vi "ATF_PUMP_PID_screen_V1.0.vi"() -> ()   [LabVIEW 2022 SP3]
panel:
  out "Countdown Timer (CDT)":dbl format="T%<+%H:%M:%S%3u>t"
  out "Date":timestamp format="%<%d/%m/%Y>T"
  in  "Close":bool
  in  "Screen No":dbl
  out "Indian Standard Time (IST)":timestamp format="%<%H:%M:%S%2u>T"
  out "B_AT_PV_19_HSS":bool
  out "B_AT_PV_19":bool caption="Boolean"
  out "B_AT_PV_18_HSS":bool
  out "B_AT_PV_18":bool caption="Boolean"
  out "B_AT_PV_16_HSS":bool
  out "B_AT_PV_16":bool caption="Boolean"
  out "B_AT_PV_14_HSS":bool
  out "B_AT_PV_14":bool caption="Boolean"
  out "B_AT_PV_12_HSS":bool
  out "B_AT_PV_12":bool caption="Boolean"
  out "B_AT_PV_10_HSS":bool
  out "B_AT_PV_10":bool caption="Boolean"
  out "B_AT_PV_08_HSS":bool
  out "B_AT_PV_08":bool caption="Boolean"
  out "B_AT_PV_06_HSS":bool
  out "B_AT_PV_06":bool caption="Boolean"
  out "B_AT_PV_04_HSS":bool
  out "B_AT_PV_04":bool caption="Boolean"
  out "B_AT_PV_02_HSS":bool
  out "B_AT_PV_02":bool caption="Boolean"
  out "B_AT_PV_17_HSS":bool
  out "B_AT_PV_17":bool caption="Boolean"
  out "B_AT_PV_15_HSS":bool
  out "B_AT_PV_15":bool caption="Boolean"
  out "B_AT_PV_13_HSS":bool
  out "B_AT_PV_13":bool caption="Boolean"
  out "B_AT_PV_11_HSS":bool
  out "B_AT_PV_11":bool caption="Boolean"
  out "B_AT_PV_09_HSS":bool
  out "B_AT_PV_09":bool caption="Boolean"
  out "B_AT_PV_07_HSS":bool
  out "B_AT_PV_07":bool caption="Boolean"
  out "B_AT_PV_05_HSS":bool
  out "B_AT_PV_05":bool caption="Boolean"
  out "B_AT_PV_03_HSS":bool
  out "B_AT_PV_03":bool caption="Boolean"
  out "B_AT_PV_01_HSS":bool
  out "B_AT_PV_01":bool caption="Boolean"
  out "S_PT_19":dbl format="%.2f bar"
  out "S_RTD_19":dbl format="%.2f bar"
  out "D_PT_19":dbl format="%.2f bar"
  out "D_RTD_19":dbl format="%.2f bar"
  out "S_PT_16":dbl format="%.2f bar"
  out "S_RTD_16":dbl format="%.2f bar"
  out "D_PT_16":dbl format="%.2f bar"
  out "D_RTD_16":dbl format="%.2f bar"
  out "S_PT_15":dbl format="%.2f bar"
  out "S_RTD_15":dbl format="%.2f bar"
  out "D_PT_15":dbl format="%.2f bar"
  out "D_RTD_15":dbl format="%.2f bar"
  out "S_PT_12":dbl format="%.2f bar"
  out "S_RTD_12":dbl format="%.2f bar"
  out "D_PT_12":dbl format="%.2f bar"
  out "D_RTD_12":dbl format="%.2f bar"
  out "S_PT_11":dbl format="%.2f bar"
  out "S_RTD_11":dbl format="%.2f bar"
  out "D_PT_11":dbl format="%.2f bar"
  out "D_RTD_11":dbl format="%.2f bar"
  out "S_PT_18":dbl format="%.2f bar"
  out "S_RTD_18":dbl format="%.2f bar"
  out "D_PT_18":dbl format="%.2f bar"
  out "D_RTD_18":dbl format="%.2f bar"
  out "S_PT_14":dbl format="%.2f bar"
  out "S_RTD_14":dbl format="%.2f bar"
  out "D_PT_14":dbl format="%.2f bar"
  out "D_RTD_14":dbl format="%.2f bar"
  out "S_PT_10":dbl format="%.2f bar"
  out "S_RTD_10":dbl format="%.2f bar"
  out "D_PT_10":dbl format="%.2f bar"
  out "D_RTD_10":dbl format="%.2f bar"
  out "S_PT_17":dbl format="%.2f bar"
  out "S_RTD_17":dbl format="%.2f bar"
  out "D_PT_17":dbl format="%.2f bar"
  out "D_RTD_17":dbl format="%.2f bar"
  out "S_PT_13":dbl format="%.2f bar"
  out "S_RTD_13":dbl format="%.2f bar"
  out "D_PT_13":dbl format="%.2f bar"
  out "D_RTD_13":dbl format="%.2f bar"
  out "S_PT_09":dbl format="%.2f bar"
  out "S_RTD_09":dbl format="%.2f bar"
  out "D_PT_09":dbl format="%.2f bar"
  out "D_RTD_09":dbl format="%.2f bar"
  out "S_PT_08":dbl format="%.2f bar"
  out "S_RTD_08":dbl format="%.2f bar"
  out "D_PT_08":dbl format="%.2f bar"
  out "D_RTD_08":dbl format="%.2f bar"
  out "S_PT_07":dbl format="%.2f bar"
  out "S_RTD_07":dbl format="%.2f bar"
  out "D_PT_07":dbl format="%.2f bar"
  out "D_RTD_07":dbl format="%.2f bar"
  out "S_PT_06":dbl format="%.2f bar"
  out "S_RTD_06":dbl format="%.2f bar"
  out "D_PT_06":dbl format="%.2f bar"
  out "D_RTD_06":dbl format="%.2f bar"
  out "S_PT_05":dbl format="%.2f bar"
  out "S_RTD_05":dbl format="%.2f bar"
  out "D_PT_05":dbl format="%.2f bar"
  out "D_RTD_05":dbl format="%.2f bar"
  out "S_PT_04":dbl format="%.2f bar"
  out "S_RTD_04":dbl format="%.2f bar"
  out "D_PT_04":dbl format="%.2f bar"
  out "D_RTD_04":dbl format="%.2f bar"
  out "S_PT_03":dbl format="%.2f bar"
  out "S_RTD_03":dbl format="%.2f bar"
  out "D_PT_03":dbl format="%.2f bar"
  out "D_RTD_03":dbl format="%.2f bar"
  out "S_PT_02":dbl format="%.2f bar"
  out "S_RTD_02":dbl format="%.2f bar"
  out "D_PT_02":dbl format="%.2f bar"
  out "D_RTD_02":dbl format="%.2f bar"
  out "S_PT_01":dbl format="%.2f bar"
  out "S_RTD_01":dbl format="%.2f bar"
  out "D_PT_01":dbl format="%.2f bar"
  out "D_RTD_01":dbl format="%.2f bar"
  out "B_AT_T_04":dbl format="%.2f bar"
  out "B_AT_T_05":dbl format="%.2f bar"
  out "B_LO_P_09":dbl format="%.2f bar"
  out "B_LO_P_10":dbl format="%.2f bar"
  # "BSTF P&ID SCREEN"
  # "VERSION 1.0"
  # "8"
  # "7"
  # "6"
  # "4"
  # "3"
  # "12"
  # "11"
  # "10"
  # "16"
  # "15"
  # "14"
  # "19"
  # "18"
  # "17"
  # "13"
  # "9"
  # "5"
  # "2"
  # "1"
  # "ATF MANIFOLD"
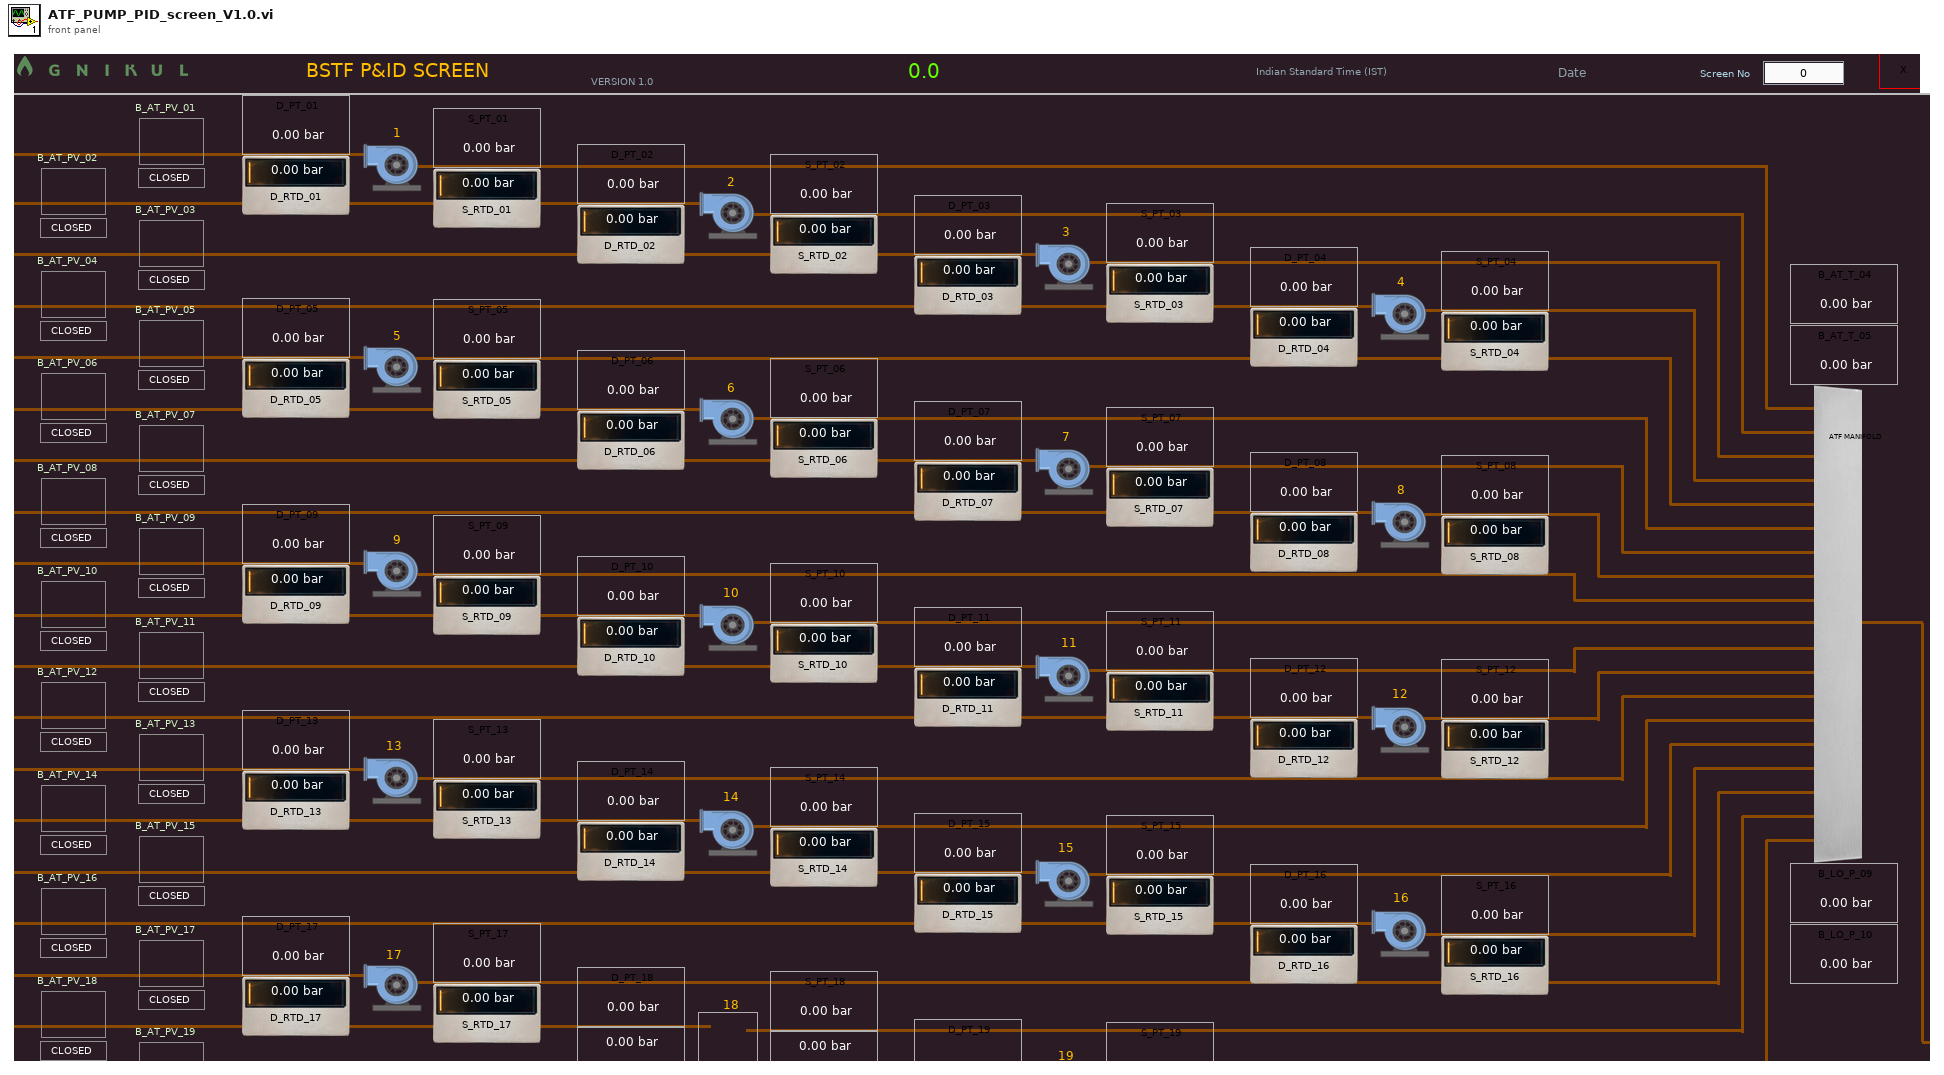
[diagram p1: front panel]
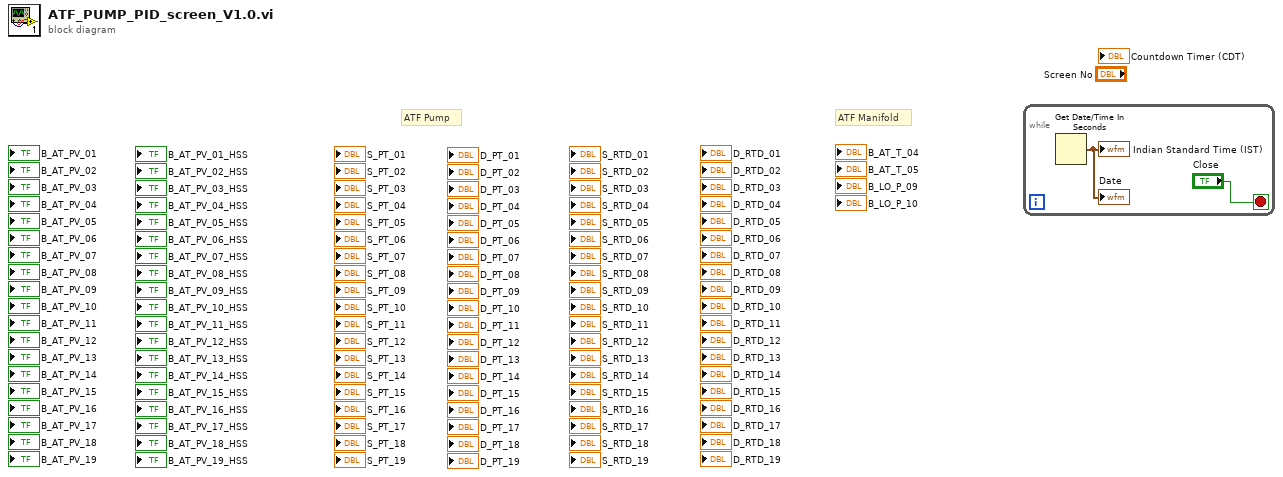
[diagram p0: block diagram]
diagram:
  # "ATF Pump"
  # "ATF Manifold"
  n1 = while {
    stop <- "Close" stop-if-true
    n2 = Get Date/Time In Seconds() -> (seconds since 1Jan1904=→"Date" →"Indian Standard Time (IST)":timestamp)
  }
